vi "stopwatch FGV.vi"(10 "error in":errorcluster, 11 "state":enum16{"Restart", "Stop"}(ring)) -> (2 "error out":errorcluster, 3 "duration (s)":dbl)   [LabVIEW 2020]
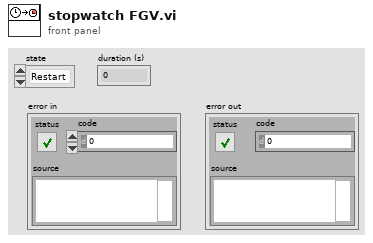
[diagram p1: front panel]
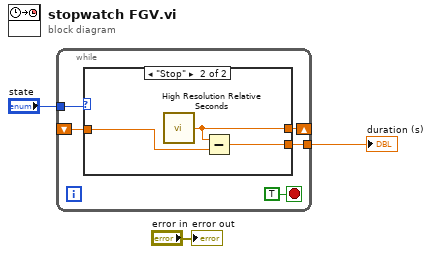
[diagram p0: block diagram]
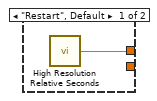
[diagram p2: hidden frame]
diagram:
  n1 = while {
    tunnel: [w8] -> w3
    shift-right: [w6] -> _
    shift-left: _ -> [w4]
    tunnel: "state" -> [w5]
    stop <- TRUE stop-if-true
    n2 = case shown="\"Stop\"" w5 {
      tunnel: [_ w12] -> w8
      tunnel: [w9 w11] -> w6
      tunnel: w4 -> [_ w10]
      frame "Restart", Default {
        n3 = call <vilib>:"High Resolution Relative Seconds.vi"() -> ("relative seconds"=w9:dbl)
      }
      frame "Stop" {
        n4 = call <vilib>:"High Resolution Relative Seconds.vi"() -> ("relative seconds"=w11:dbl)
        n5 = Subtract(x=w11, y=w10) -> (x-y=w12:dbl)
      }
    }
  }
  "duration (s)" <- w3
  "error out" <- "error in"
